vi "Wait Time (mSec).vi"(8 "error in":errorcluster, 11 "Spin Amount (mS)":u32) -> (0 "error out":errorcluster)   [LabVIEW 2023]
doc: "Consumes the processor for Spin Amount (ms), allowing the user to easily introduce lateness into a loop."
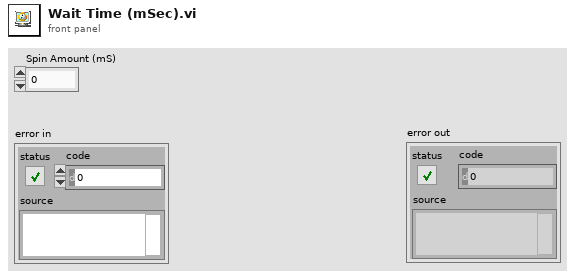
[diagram p1: front panel]
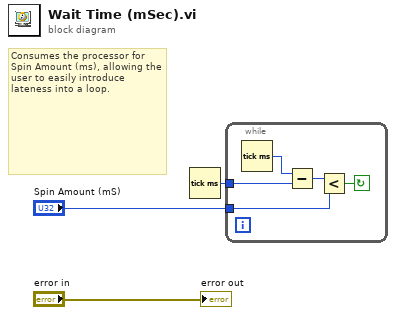
[diagram p0: block diagram]
diagram:
  # "Consumes the processor for Spin Amount (ms), allowing the user to easily introduce lateness into a loop."
  n1 = Tick Count (ms)() -> (millisecond timer value=w3:u32)
  n2 = while {
    tunnel: "Spin Amount (mS)" -> [w4]
    tunnel: w3 -> [w7]
    stop <- w5 continue-if-true
    n3 = Tick Count (ms)() -> (millisecond timer value=w8:u32)
    n4 = Subtract(x=w8, y=w7) -> (x-y=w6:u32)
    n5 = Less?(x=w6, y=w4) -> (x < y?=w5:bool)
  }
  "error out" <- "error in"
